vi "Fetch Measurement (Carrier Power - Frequency).vi"(8 "error in (no error)":errorcluster, 11 "VISA resource name":refnum<visa-resource-name>) -> (0 "error out":errorcluster, 1 "Carrier Frequency (Hz)":dbl, 2 "Carrier Power (dBm)":dbl, 3 "VISA resource name out":refnum<visa-resource-name>)   [LabVIEW 2014, in "Agilent ESA PSA Series.lvlib"]
doc: "Returns the results of the last measurement (Carrier Power and Frequency) and does not initiate data acquisition.\n\n<B>Note:</B>\n\n This VI is valid for both Spot Frequency and Log Plot functionalities of the Phase Noise personality."
uses:
  Agilent ESA PSA Series.lvlib
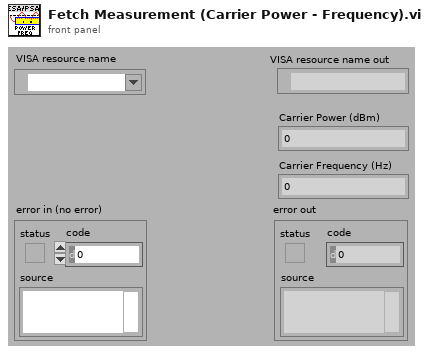
[diagram p1: front panel]
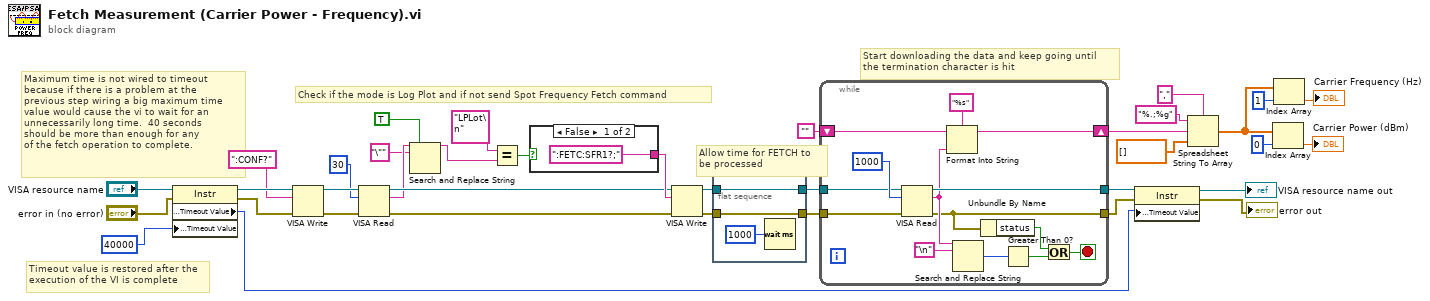
[diagram p0: block diagram]
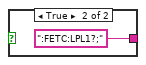
[diagram p2: hidden frame]
diagram:
  # "Maximum time is not wired to timeout\nbecause if there is a problem at the\nprevious step wiring a big maximum time\nvalue would cause the vi to wait for an\nunnecessarily long time.  40 seconds\nshould be more than enough for any\nof the fetch operation to complete."
  # "Timeout value is restored after the\nexecution of the VI is complete"
  # "Start downloading the data and keep going until\nthe termination character is hit"
  # "Allow time for FETCH to\nbe processed"
  # "Check if the mode is Log Plot and if not send Spot Frequency Fetch command"
  n1 = property on="Property Node" class="Instr"(reference="VISA resource name", error in="error in (no error)", "General Settings:Timeout Value"=u32 40000) -> (reference out=w34:refnum<visa-resource-name>, error out=w35:errorcluster, "General Settings:Timeout Value"=w31:u32)
  n2 = VISA Write(VISA resource name=w34, write buffer=":CONF?", error in (no error)=w35) -> (VISA resource name out=w17:refnum<visa-resource-name>, error out=w16:errorcluster)  [unwired: 1 out]
  n3 = VISA Read(VISA resource name=w17, byte count=u32 30, error in (no error)=w16) -> (VISA resource name out=w13:refnum<visa-resource-name>, read buffer=w9:string, error out=w12:errorcluster)  [unwired: 1 out]
  n4 = Search and Replace String(replace all?=TRUE ("replace all? (F)"), input string=w9, search string="\"") -> (result string=w6:string)  [unwired: 5 in, 3 out]
  n5 = Equal?(x="LPLot\n", y=w6) -> (x = y?=w11:bool)
  n6 = case shown="False" w11 {
    tunnel: [":FETC:SFR1?;" ("string (\"\")") ":FETC:LPL1?;" ("string (\"\")")] -> w14
    frame False {
    }
    frame True {
    }
  }
  n7 = VISA Write(VISA resource name=w13, write buffer=w14, error in (no error)=w12) -> (VISA resource name out=w4:refnum<visa-resource-name>, error out=w5:errorcluster)  [unwired: 1 out]
  n8 = flat-sequence {
    tunnel: w5 -> [w41]
    tunnel: w4 -> [w42]
    tunnel: [w42] -> w2
    tunnel: [w41] -> w3
    frame #0 {
      n9 = Wait (ms)(milliseconds to wait=u32 1000) -> ()  [unwired: 1 out]
    }
  }
  n10 = while {
    tunnel: [w55] -> w33
    tunnel: [w46] -> w32
    tunnel: w2 -> [w54]
    tunnel: w3 -> [w53]
    shift-right: [w49] -> w24
    shift-left: "" -> [w48]
    stop <- w44 stop-if-true
    n11 = VISA Read(VISA resource name=w54, byte count=u32 1000, error in (no error)=w53) -> (VISA resource name out=w55:refnum<visa-resource-name>, read buffer=w50:string, error out=w46:errorcluster)  [unwired: 1 out]
    n12 = Format Into String(format string="%s", initial string=w48, w50) -> (resulting string=w49:string)  [unwired: 1 in, 1 out]
    n13 = Search and Replace String(input string=w50, search string="\n") -> (number of replacements=w51:i32)  [unwired: 6 in, 3 out]
    n14 = Unbundle By Name(w46) -> ("status"=w43:bool)
    n15 = Greater Than 0?(x=w51) -> (x > 0?=w45:bool)
    n16 = Or(x=w43, y=w45) -> (x .or. y?=w44:bool)
  }
  n17 = property on="Property Node" class="Instr"(reference=w33, error in=w32, "General Settings:Timeout Value"=w31) -> (reference out=→"VISA resource name out":refnum<visa-resource-name>, error out=→"error out":errorcluster)
  n18 = Spreadsheet String To Array(delimiter (Tab)=",", format string="%.;%g", spreadsheet string=w24, array type (2D Dbl)=dbl[] []) -> (array=w22:dbl[])
  n19 = Index Array(array=w22, index=0) -> (element=→"Carrier Power (dBm)":dbl)
  n20 = Index Array(array=w22, index=1) -> (element=→"Carrier Frequency (Hz)":dbl)
